vi "Get Value.vi"(8 "error in (no error)":errorcluster, 10 "name":string, 11 "Keyed Value Tree in":refnum<class "Keyed Value Tree.lvclass">) -> (0 "error out":errorcluster, 1 "value":string, 2 "found":bool, 3 "Keyed Value Tree out":refnum<class "Keyed Value Tree.lvclass">)   [LabVIEW 2027, in "Keyed Value Tree.lvclass"]
uses:
  Keyed Value Tree.lvclass
  Keyed Value Tree.lvclass/Keyed Value Tree.ctl
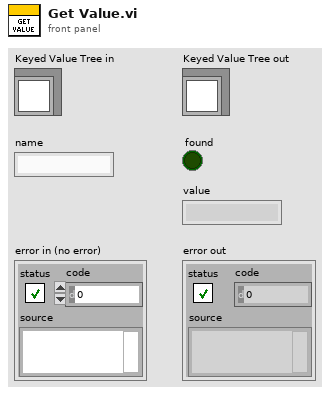
[diagram p1: front panel]
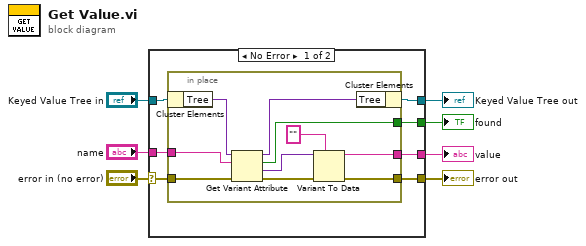
[diagram p0: block diagram]
diagram:
  n1 = case shown="No Error" "error in (no error)" {
    selector: "error in (no error)" -> [w11 w26]
    tunnel: [w10 w26] -> w5
    tunnel: [w13 w25] -> w6
    tunnel: "Keyed Value Tree in" -> [w14 w25]
    tunnel: [w12 _] -> w2
    tunnel: "name" -> [w9 _]
    tunnel: [w8 _] -> w1
    frame No Error {
      n2 = in-place {
        in-place-border: [w22] -> w12
        in-place-border: w11 -> [w21]
        in-place-border: [w15] -> w10
        in-place-border: w9 -> [w20]
        in-place-border: [w17] -> w8
        n3 = in-place-cluster #1(w14) -> ("Tree"=w24:variant)
        n4 = Get Variant Attribute(Variant=w24, name=w20, error in=w21) -> (duplicate Variant=w23:variant, found=w22:bool, value=w19:variant, error out=w16:errorcluster)  [unwired: 1 in]
        n5 = Variant To Data(error in=w16, type="" ("name 3"), Variant=w19) -> (data=w17:string, error out=w15:errorcluster)
        n6 = in-place-cluster #1("Tree"=w23) -> (w13:refnum<class "Keyed Value Tree.lvclass">)
      }
    }
    frame Error {
    }
  }
  "error out" <- w5
  "Keyed Value Tree out" <- w6
  "found" <- w2
  "value" <- w1
